vi "MoveLineROI.vi"(7 "Action":enum16{"X+", "X-", "Y+", "Y-"}(ring), 8 "error in (no error)":errorcluster, 9 "PItch":i32, 10 "ROI In":T1 {"Contours"."Type" items=["No Selection", "Point", "Line", "Rectangle", "Oval", "Polygon", "Freehand Region", "Annulus", "Unused2", "Unused3", "Broken Line", "Freehand Line", "Rotated Rectangle"]}) -> (0 "error out":errorcluster, 2 "ROI Out":T1 {"Contours"."Type" items=["No Selection", "Point", "Line", "Rectangle", "Oval", "Polygon", "Freehand Region", "Annulus", "Unused2", "Unused3", "Broken Line", "Freehand Line", "Rotated Rectangle"]})   [LabVIEW 2019]
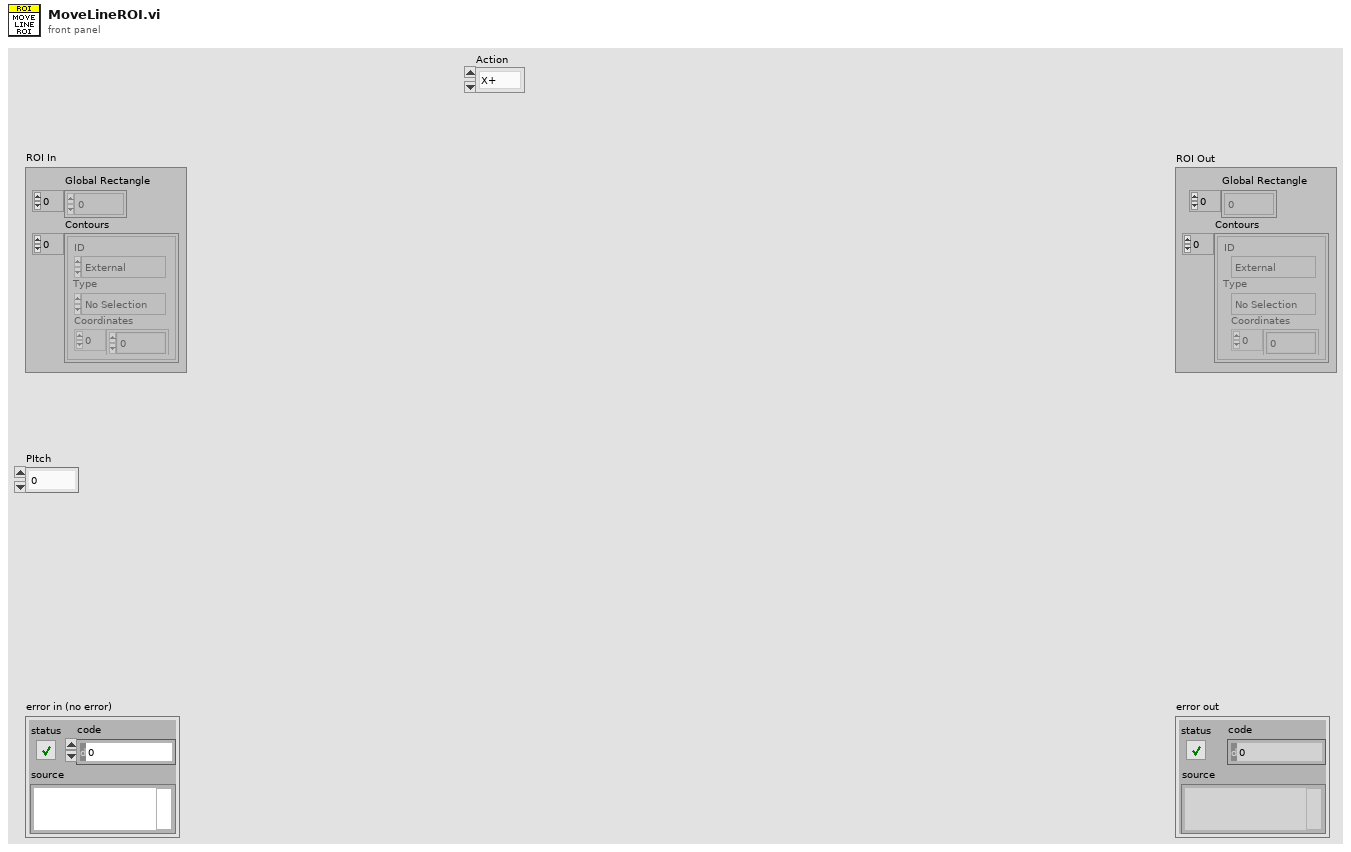
[diagram p1: front panel]
types:
  T1 = typedef "ROI Descriptor" = cluster{"Global Rectangle":i32[], "Contours":cluster{"ID":enum32{"External", "Internal"}, "Type":u32, "Coordinates":i32[]}[]}
  T2 = typedef "IMAQ Line" = cluster{"Start X":i32, "Start Y":i32, "End X":i32, "End Y":i32}
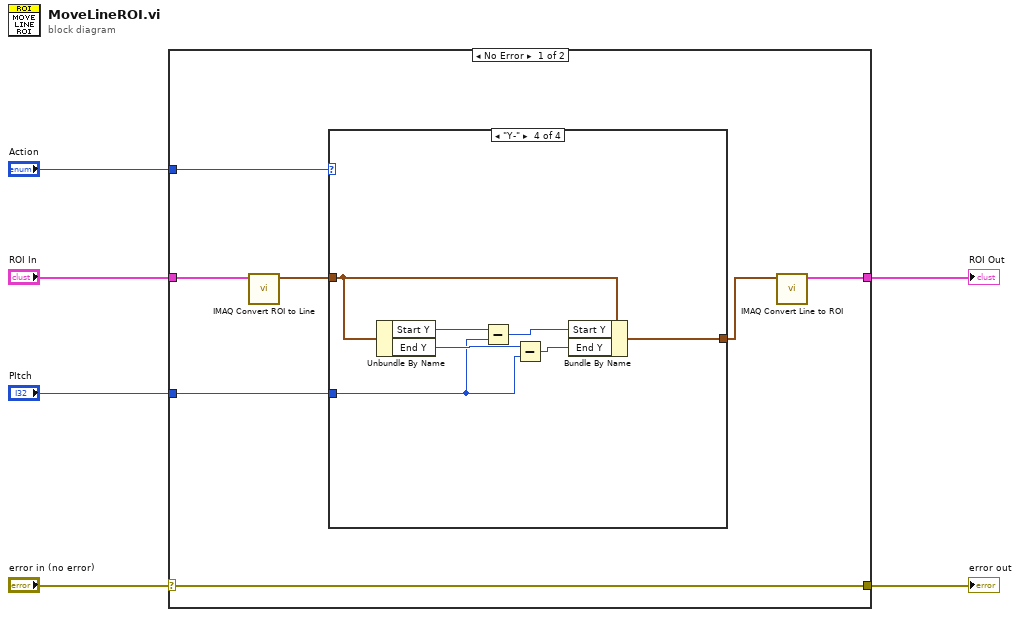
[diagram p0: block diagram]
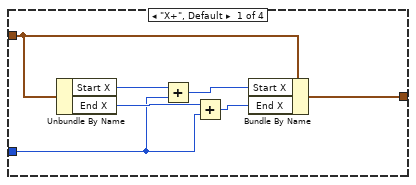
[diagram p2: hidden frame]
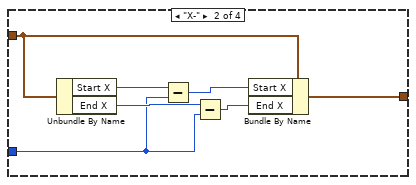
[diagram p3: hidden frame]
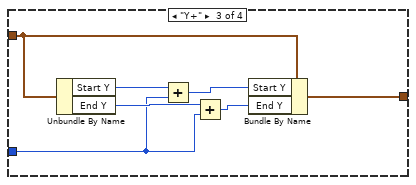
[diagram p4: hidden frame]
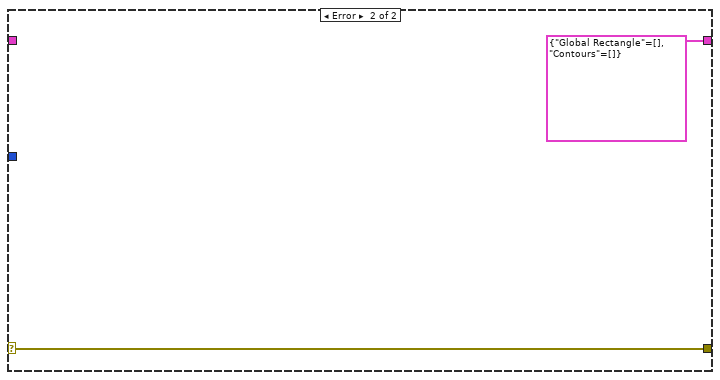
[diagram p5: hidden frame]
diagram:
  n1 = case shown="No Error" "error in (no error)" {
    selector: "error in (no error)" -> [w10 w43]
    tunnel: [w10 w43] -> w5
    tunnel: "Action" -> [w13 _]
    tunnel: "PItch" -> [w12 _]
    tunnel: [w9 T1 {"Global Rectangle"=[], "Contours"=[]} ("ROI Descriptor")] -> w2
    tunnel: "ROI In" -> [w7 _]
    frame No Error {
      n2 = call "IMAQ Convert ROI to Line"("ROI Descriptor"=w7) -> ("Line"=w8:T2)  [unwired: 8 in, 1 out]
      n3 = case shown="\"Y-\"" w13 {
        tunnel: w8 -> [w15 w27 w29 w41]
        tunnel: w12 -> [w16 w22 w30 w36]
        tunnel: [w14 w21 w28 w35] -> w11
        frame "X+", Default {
          n4 = Unbundle By Name(w15) -> ("Start X"=w20:i32, "End X"=w18:i32)
          n5 = Add(x=w20, y=w16) -> (x+y=w19:i32)
          n6 = Add(x=w18, y=w16) -> (x+y=w17:i32)
          n7 = Bundle By Name(cluster=w15, "Start X"=w19, "End X"=w17) -> (w14:T2)
        }
        frame "X-" {
          n8 = Unbundle By Name(w27) -> ("Start X"=w26:i32, "End X"=w24:i32)
          n9 = Subtract(x=w26, y=w22) -> (x-y=w25:i32)
          n10 = Subtract(x=w24, y=w22) -> (x-y=w23:i32)
          n11 = Bundle By Name(cluster=w27, "Start X"=w25, "End X"=w23) -> (w21:T2)
        }
        frame "Y+" {
          n12 = Unbundle By Name(w29) -> ("Start Y"=w34:i32, "End Y"=w32:i32)
          n13 = Add(x=w34, y=w30) -> (x+y=w33:i32)
          n14 = Add(x=w32, y=w30) -> (x+y=w31:i32)
          n15 = Bundle By Name(cluster=w29, "Start Y"=w33, "End Y"=w31) -> (w28:T2)
        }
        frame "Y-" {
          n16 = Unbundle By Name(w41) -> ("Start Y"=w40:i32, "End Y"=w38:i32)
          n17 = Subtract(x=w40, y=w36) -> (x-y=w39:i32)
          n18 = Subtract(x=w38, y=w36) -> (x-y=w37:i32)
          n19 = Bundle By Name(cluster=w41, "Start Y"=w39, "End Y"=w37) -> (w35:T2)
        }
      }
      n20 = call "IMAQ Convert Line to ROI"("Line"=w11) -> ("ROI Descriptor"=w9:T1)  [unwired: 8 in, 1 out]
    }
    frame Error {
    }
  }
  "error out" <- w5
  "ROI Out" <- w2
